vi "startUp.vi"(8 "error in (no error)":errorcluster, 11 "ImageStreamViewer in":refnum<class "ImageStreamViewer.lvclass">) -> (0 "error out":errorcluster, 3 "ImageStreamViewer out":refnum<class "ImageStreamViewer.lvclass">)   [LabVIEW 2009, in "Views.lvlib" / "Camera.lvlib" / "ImageStreamViewer.lvclass"]
uses:
  ImageStreamViewer.lvclass
  Tools/ImageProcessor/ImageAnalyser/FluorescenceAnalyser/FluorescenceAnalyser.lvclass
  ImageStreamViewer.lvclass/ImageStreamViewer.ctl
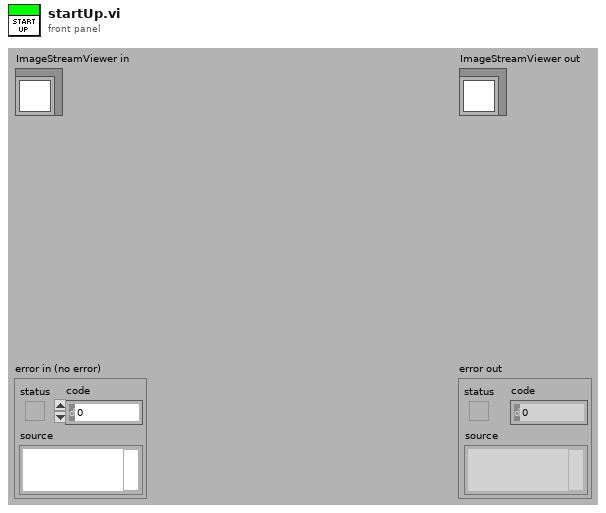
[diagram p1: front panel]
types:
  T1 = typedef "Image Type" = u32
  T2 = typedef "IMAQ Image.ctl" = refnum<image>
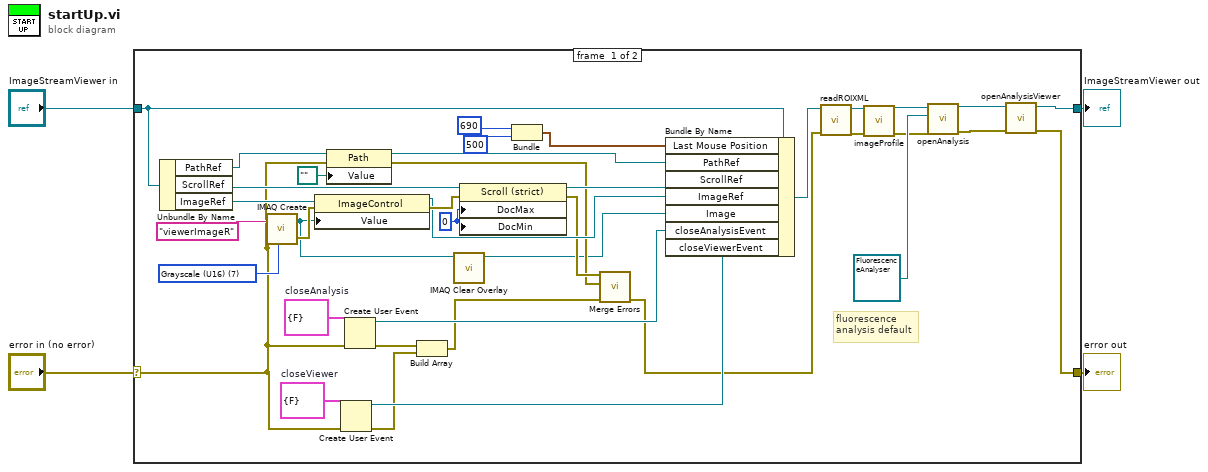
[diagram p0: block diagram]
diagram:
  n1 = case shown="No Error" "error in (no error)" {
    selector: "error in (no error)" -> [w22 w45]
    tunnel: [w14 w45] -> w3
    tunnel: [w17 w44] -> w1
    tunnel: "ImageStreamViewer in" -> [w34 w44]
    frame #0 {
      w23 = cluster{"close":bool} {"close"=FALSE}  # closeViewer
      w28 = cluster{"close":bool} {"close"=FALSE}  # closeAnalysis
      w37 = 0
      w43 = T1 7 items=["Grayscale (U8)", "Grayscale (I16)", "Grayscale (SGL)", "Complex (CSG)", "RGB (U32)", "HSL (U32)", "RGB (U64)", "Grayscale (U16)"] ("Image Type")
      # "fluorescence \nanalysis default"
      n2 = Unbundle By Name(w34) -> ("PathRef"=w33:refnum<vi>, "ScrollRef"=w39:refnum<vi>, "ImageRef"=w40:refnum<vi>)
      n3 = call "IMAQ Create"("Image Name"="viewerImageR", "Image Type"=w43, "error in (no error)"=w22) -> ("New Image"=w6:T2, "error out"=w41:errorcluster)  [unwired: 2 in]
      n4 = property class="ImageControl"(reference=w40, error in=w41, "Value"=w6) -> (reference out=w35:refnum<vi>, error out=w38:errorcluster)
      n5 = property class="Path"(reference=w33, error in=w22, "Value"=path "") -> (reference out=w29:refnum<vi>, error out=w30:errorcluster)
      n6 = Create User Event(user event datatype=w23, error in=w22) -> (user event=w21:refnum<user-event>, error out=w19:errorcluster)
      n7 = Create User Event(user event datatype=w28, error in=w22) -> (user event=w27:refnum<user-event>, error out=w20:errorcluster)
      n8 = Build Array(w20, w19) -> (w18:errorcluster[])
      n9 = call "IMAQ Clear Overlay"("Image"=w6) -> ("Image Out"=w5:T2)  [unwired: 9 in, 1 out]
      n10 = property class="Scroll (strict)"(reference=w39, error in=w38, "DocMax"=w37, "DocMin"=w37) -> (reference out=w36:refnum<vi>, error out=w31:errorcluster)
      n11 = Bundle(690, 500) -> (w24:cluster{i32, i32})  [unwired: 1 in]
      n12 = call <vilib>:"Merge Errors.vi"("error array in"=w18, "error in 2 (no error)"=w30, "error in 1 (no error)"=w31) -> ("error out"=w11:errorcluster)  [unwired: 4 in]
      n13 = Bundle By Name(cluster=w34, "Last Mouse Position"=w24, "PathRef"=w29, "ScrollRef"=w36, "ImageRef"=w35, "Image"=w5, "closeAnalysisEvent"=w27, "closeViewerEvent"=w21) -> (w12:refnum<class "ImageStreamViewer.lvclass">)
      n14 = call "readROIXML.vi"("error in (no error)"=w11, "ImageStreamViewer in"=w12) -> ("error out"=w9:errorcluster, "ImageStreamViewer out"=w10:refnum<class "ImageStreamViewer.lvclass">)  [unwired: 8 in]
      n15 = call "imageProfile.vi"("error in (no error)"=w9, "ImageStreamViewer in"=w10) -> ("error out"=w7:errorcluster, "ImageStreamViewer out"=w8:refnum<class "ImageStreamViewer.lvclass">)  [unwired: 8 in]
      n16 = call "openAnalysis.vi"("error in (no error)"=w7, "ImageAnalyser"=refnum<class "FluorescenceAnalyser.lvclass"> refnum ("Tools.lvlib:Imaging.lvlib:FluorescenceAnalyser.lvclass"), "ImageStreamViewer in"=w8) -> ("error out"=w15:errorcluster, "ImageStreamViewer out"=w16:refnum<class "ImageStreamViewer.lvclass">)  [unwired: 7 in]
      n17 = call "openAnalysisViewer.vi"("error in (no error)"=w15, "ImageStreamViewer in"=w16) -> ("error out"=w14:errorcluster, "ImageStreamViewer out"=w17:refnum<class "ImageStreamViewer.lvclass">)  [unwired: 8 in]
    }
    frame #1 {
    }
  }
  "error out" <- w3
  "ImageStreamViewer out" <- w1
